vi "CreateBaseParentObject.vi"() -> (3 "baseParentClass out":refnum<class "baseParentClass.lvclass">)   [LabVIEW 2011, in "baseParentClass.lvclass"]
uses:
  baseParentClass.lvclass
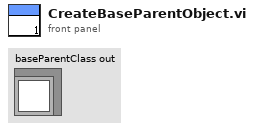
[diagram p1: front panel]
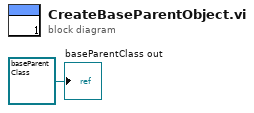
[diagram p0: block diagram]
diagram:
  "baseParentClass out" <- refnum<class "baseParentClass.lvclass"> refnum ("baseParentClass out")
